vi "Get Nested Object Item by Name Array.vi"(7 "Item Path (as array of names)":string[](array[string]), 8 "error in (no error)":errorcluster, 10 "Object Offset":i32, 11 "JSON":string) -> (0 "error out":errorcluster, 1 "Offset past Item (or past last Item, if not found)":i32, 2 "Item Offset (-1 if not found)":i32, 3 "Found":bool)   [LabVIEW 2013, in "JSONtext.lvlib"]
uses:
  JSONtext.lvlib
  support/JSONtext support.lvlib
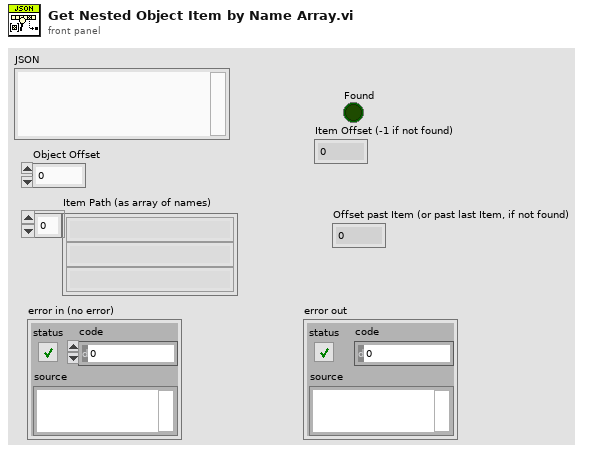
[diagram p1: front panel]
types:
  T1 = typedef "JSONtext.lvlib/JSON Value Search.ctl" = enum16{"Parser Error", "In Object", "In Array", "String", "Number", "Leading Whitespace", "Object end", "Array end", "Value end", "Undefined"}
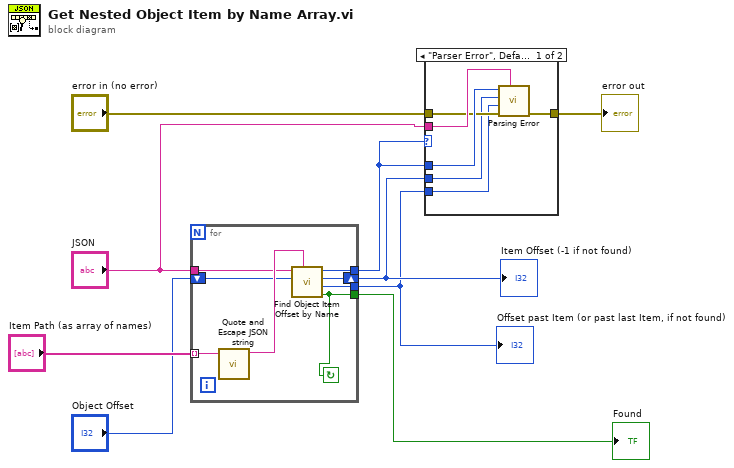
[diagram p0: block diagram]
diagram:
  n1 = for {
    tunnel: [w10] -> w9
    tunnel: [w17] -> w8
    tunnel: "JSON" -> [w15]
    tunnel: [w13] -> w3
    tunnel: "Item Path (as array of names)" -> [w12] mode=indexing
    shift-right: [w14] -> w4
    shift-left: "Object Offset" -> [w11]
    stop <- w10 continue-if-true
    n2 = call "Quote and Escape JSON string.vi"("Plain Text"=w12) -> ("<JSON>"=w16:string)  [unwired: 10 in]
    n3 = call "Find Object Item Offset by Name.vi"("Item Name <JSON>"=w16, "Object Offset"=w11, "JSON"=w15) -> ("Found"=w10:bool, "Offset past Item (or past last Item, if not found)"=w13:i32, "Item Offset (-1 if not found)"=w14:i32, "State"=w17:T1)  [unwired: 4 in, 1 out]
  }
  "Found" <- w9
  "Item Offset (-1 if not found)" <- w4
  "Offset past Item (or past last Item, if not found)" <- w3
  n4 = case shown="\"Parser Error\", Default" w8 {
    tunnel: w8 -> [w23 _]
    tunnel: "JSON" -> [w22 _]
    tunnel: "error in (no error)" -> [w21 w24]
    tunnel: [w20 w24] -> w6
    tunnel: w4 -> [w19 _]
    tunnel: w3 -> [w18 _]
    frame "Parser Error", Default {
      n5 = call "Parsing Error.vi"("JSON"=w22, "error in (no error)"=w21, "Offset past match"=w18, "Value start"=w19, "State"=w23) -> ("error out"=w20:errorcluster)  [unwired: 6 in]
    }
    frame "Value end" {
    }
  }
  "error out" <- w6
